vi "Piston Hold.vi"(1 "Input":bool, 2 "Invert?":bool) -> (0 "Output":T1)   [LabVIEW 2020, in "TitanLib.lvlib"]
uses:
  <vilib>/Rock Robotics/WPI/Solenoid/WPI_SolenoidValue.ctl
  TitanLib.lvlib
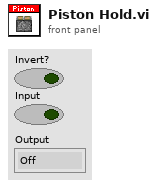
[diagram p1: front panel]
types:
  T1 = typedef "WPI_SolenoidValue.ctl" = enum16{"Off", "On", "Forward", "Reverse"}
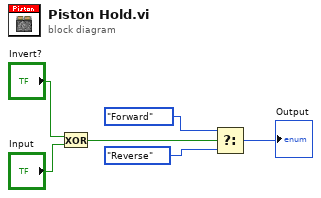
[diagram p0: block diagram]
diagram:
  n1 = Exclusive Or(1:"Input", 2:"Invert?") -> (0:w1:bool)
  n2 = Select(t=WPI_SolenoidValue."Forward" ("Value"), s=w1, f=WPI_SolenoidValue."Reverse" ("Value")) -> (s? t:f=→"Output":T1)
